vi "FP_Size to GObject.vi"(6 "Border Spacing (2 Px)":i32, 7 "Calling VI's Ref":refnum<vi>, 8 "Error":errorcluster, 11 "GObj Refnum":refnum<vi>) -> (0 "Error Out":errorcluster, 2 "Front Panel.PanelBounds Out":T1, 3 "GObj Refnum Out":refnum<vi>, 5 "Calling VI's Ref Out":refnum<vi>)   [LabVIEW 2020]
doc: "Sizes the VI Window to the GObject"
uses:
  <vilib>/Utility/miscctls.llb/LVRectTypeDef.ctl
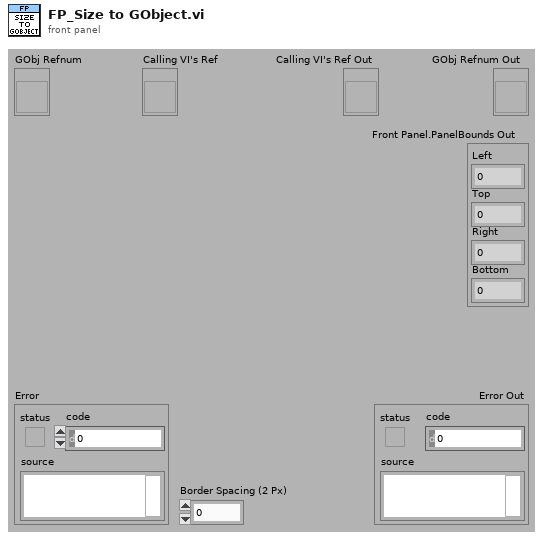
[diagram p1: front panel]
types:
  T1 = typedef "LVRectTypeDef.ctl" = cluster{"Left":i16, "Top":i16, "Right":i16, "Bottom":i16}
  T2 = typedef "LVPositionTypeDef.ctl" = cluster{"Left":i32, "Top":i32}
  T3 = typedef "LVBoundsTypeDef.ctl" = cluster{"Width":u32, "Height":u32}
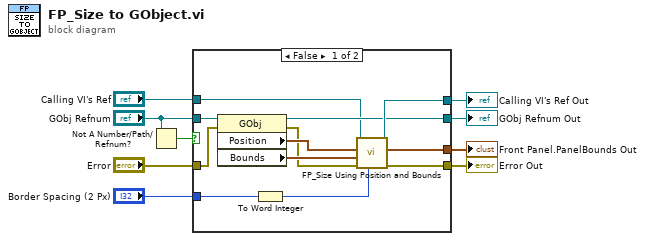
[diagram p0: block diagram]
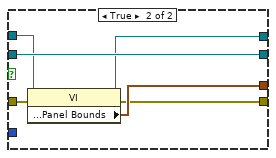
[diagram p2: hidden frame]
diagram:
  n1 = Not A Number/Path/Refnum?(number/path/refnum="GObj Refnum") -> (NaN/Path/Refnum?=w1:bool)
  n2 = case shown="False" w1 {
    tunnel: [w21 w24] -> w9
    tunnel: [w12 w27] -> w8
    tunnel: "Error" -> [w20 w25]
    tunnel: [w19 w26] -> w6
    tunnel: [w17 w22] -> w5
    tunnel: "Border Spacing (2 Px)" -> [w16 _]
    tunnel: "Calling VI's Ref" -> [w11 w23]
    tunnel: "GObj Refnum" -> [w15 w27]
    frame False {
      n3 = property class="GObj"(reference=w15, error in=w20) -> (reference out=w12:refnum<vi>, error out=w10:errorcluster, "Position"=w14:T2, "Bounds"=w13:T3)
      n4 = To Word Integer(number=w16) -> (16bit integer=w18:i16)
      n5 = call "FP_Size Using Position and Bounds.vi"("Border Spacing"=w18, "Error"=w10, "Bounds"=w13, "Position"=w14, "VI"=w11) -> ("Error Out"=w21:errorcluster, "Front Panel Box Out"=w19:T1, "VI Out"=w17:refnum<vi>)  [unwired: 4 in]
    }
    frame True {
      n6 = property on="Property Node" class="VI"(reference=w23, error in=w25) -> (reference out=w22:refnum<vi>, error out=w24:errorcluster, "Front Panel Window:Panel Bounds"=w26:T1)
    }
  }
  "Error Out" <- w9
  "GObj Refnum Out" <- w8
  "Front Panel.PanelBounds Out" <- w6
  "Calling VI's Ref Out" <- w5
